vi "dataAcq_get_spectrum_trace.vi"(0 "reference":refnum<class "OSA.lvclass">, 2 "spectrum trace index":u32, 5 "error in (no error)":errorcluster, 7 "spectrum trace set name":string, 9 "parameter trace set comment":string) -> (14 "duplicate reference":refnum<class "OSA.lvclass">, 19 "error out":errorcluster)   [LabVIEW 2010, in "OSA.lvclass"]
doc: "Reads data from spectrometer and updates a spectrum trace Y array, X is either equidistant, (x min and max), or a full X-array - see traces_xValueFormat.vi. The trace data buffer is allocated by FTSLib.dll during labview driver initialisation.\n\nX: periods/cm\nY: mW absolute pwr, (pwr/resolution)"
uses:
  OSA.lvclass
  typeDef/trace_properties_string.ctl
  OSA20X_misc.lvlib
  FTSLib.dll
panel:
  in  "parameter":T1=enum."name [max 32]"
  in  "length":u32
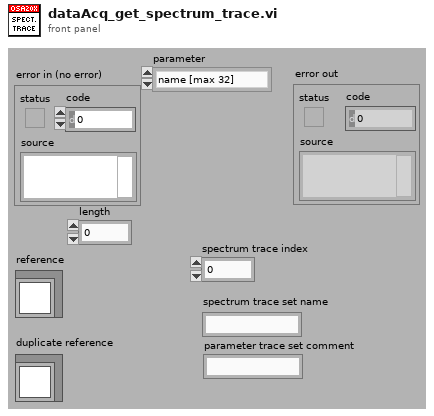
[diagram p1: front panel]
types:
  T1 = typedef "OSA.lvclass/trace_properties_string.ctl" = enum16{"interferometerSerial [max 32]", "name [max 32]", "comment [max 128]", "source [max 24]", "instr_operator [max 24]", "instr_model_str [max 24]", "all_stringParameters"}
  T2 = typedef "OSA.lvclass/ObjectAttributes.ctl" = cluster{"Stop":bool, "dataType":T3, "spectrometerIdx":u16, "buffer size interferogram":i32, "interferogram":cluster{"new":bool, "plot_x_ min":sgl, "plot_x_max":sgl, "plot_y_min":sgl, "plot_y_max":sgl, "Graph Intrfrgrm":T4, "timeStamp":u32, "signal (%)":dbl, "traces":cluster{"idx":u32, "broadBand":bool, "monoChromatic":bool, "peakToPeakSignal":dbl, "peakToPeakPos":dbl}[], "traces idx last":i32}, "spectrum":cluster{"new":bool, "plot_x_min":sgl, "plot_x_max":sgl, "plot_unit_x":T5, "plot_unit_y":T6, "plot_y_min":sgl, "plot_y_max":sgl, "Graph Spectrum":T4, "timeStamp":u32, "X_VAL_OPTIONS":enum16{"MIN_MAX", "ARRAY"}, "traces":cluster{"idx":u32}[], "traces idx last":i32}, "Thorlabs_OSA_64.lvclass:queue_action.ctlqueue ref":refnum<queue>, "action":T7, "plot zoom step":dbl, "buffer semaphore":T8, "acq stopped":bool, "dataType active":T3, "temperature (degr C)":sgl, "pressure (hPa)":sgl, "rel humidity (%)":sgl, "settings":cluster{"resolution":T9, "sensitivity":T10, "Average":bool, "average nr":u32, "apodisation":T11, "acq delay (ms)":u32, "airMesure":T12, "wmtr on":bool, "intfgrm_smooth_width":u16, "intfgrm_smooth_nrOfPasses":u16, "intfgrm_smooth":T13, "phaseCorrection":T14, "zeroFill":u8, "spectr_smooth":T13, "spectr_smooth_width":u16, "spectr_smooth_nrOfPasses":u16, "resolution (/cm)":sgl, "REF wavelength, (nm)":dbl, "gain_idx":u16, "gainAuto":bool, "gain_relative":dbl, "PD sensitivity mode":T15, "PD senseMode implemented":bool, "SensorTemperature implemented":bool, "SensorPressure implemented":bool, "SensorHumidity implemented":bool}, "peaks position":sgl[], "peaks width":sgl[], "peaks height":sgl[], "peaks max nr":u32, "peaks latest nr":i32, "peaks new":bool, "power":dbl, "power new":bool, "path":string, "wavelength (WNr)":dbl, "wavelength new":bool, "buffer size spectrum":i32, "status":string, "VI reference":refnum<vi>, "funcPointer":u64, "libraryPointer":u64, "singleAcquisition":bool, "coherenceLength (cm)":dbl, "coherenceLength new":bool, "spectrometer model":string, "spectrometer serial nr":string, "peaks thld left":sgl[], "peaks thld right":sgl[], "coherenceLength error (cm)":dbl, "ADC bits":u16, "peaks position centroid":sgl[], "peaks height centroid":sgl[], "OSA series":T16, "channel index spectrum":u16, "spectrometer rangeLow, (/cm)":dbl, "spectrometer rangeHigh, (/cm)":dbl, "channel index interferogram":u16}
  T3 = typedef "OSA.lvclass/acq_dataType.ctl" = enum16{"none", "interferogram", "spectrum"}
  T4 = typedef "OSA.lvclass/graph_intensity.ctl" = refnum<vi>
  T5 = typedef "OSA.lvclass/spectrum_x_unit.ctl" = enum16{"wavenr/cm", "THz", "eV", "nm_air", "nm_vac"}
  T6 = typedef "OSA.lvclass/y_unit.ctl" = enum16{"ADC counts", "dBm pwr absolute", "dBm pwr density", "mW pwr absolute", "mW pwr density"}
  T7 = typedef "OSA.lvclass/queue_action.ctl" = enum16{"none", "stop", "GUI_plotInterferogram", "GUI_plotSpectrum", "GUI_plotInterferogramRescale", "GUI_plotSpectrumRescale", "GUI_plotInterferogramReset", "GUI_plotSpectrumReset", "GUI_plotInterferogramAutoScaleY", "GUI_plotSpectrumAutoScaleY", "GUI_plotInterferogramZoomOut", "GUI_plotSpectrumZoomOut", "GUI_plotInterferogramPane", "GUI_plotSpectrumPane", "GUI_plotInterferogramZoomMouse", "GUI_plotSpectrumZoomMouse", "ENVIRONMENT temperature", "ENVIRONMENT pressure", "MODE_resolution set", "MODE_resolution get", "MODE_sensitivity set", "MODE_sensitivity get", "MODE_PDTemperature set", "MODE_PDTemperature get", "REBOOT/RESET firmware", "ACQASYNC_acquireSingleSpectrum", "ACQASYNC_continuous start", "ACQASYNC_continuous stop\n", "ACQASYNC_get last interferogram", "ACQASYNC_get last spectrum", "ACQASYNC_get last waveNr", "ACQOPT_interferogram smoothing set", "ACQOPT_interferogram smoothing get", "ACQOPT_spectrum smoothing set", "ACQOPT_spectrum smoothing get", "ACQOPT_apodisation type set", "ACQOPT_apodisation type get", "ACQOPT_phase correction type set", "ACQOPT_phase correction type get", "ACQOPT_acqIntervall_set", "ACQOPT_acqIntervall_get", "ACQOPT_average spectrum set", "ACQOPT_average spectrum get", "ACQOPT_rolling average set", "ACQOPT_rolling average get", "ACQOPT_zero fill factor set", "ACQOPT_zero fill factor get", "ACQOPT_cycle counting set", "ACQOPT_cycle counting get", "ACQOPT_air measure option set", "ACQOPT_air measure option get", "ACQOPT_gainLevel auto get", "ACQOPT_gainLevel auto set", "ACQOPT_gainLevel get", "ACQOPT_gainLevel set", "ACQOPT_getAll", "INSTRUMENT_PROPERTY_range_WaveNr_min", "INSTRUMENT_PROPERTY_range_WaveNr_max", "INSTRUMENT_PROPERTY_reference_wavelength_cm^-1", "INSTRUMENT_PROPERTY_samplesPerRefPeriod", "INSTRUMENT_PROPERTY_resolution_waveNrPercm", "INSTRUMENT_PROPERTY_availableGainLevels", "INSTRUMENT_PROPERTY_status", "CONVERT", "ANALYSE_POWER", "ANALYSE_PEAKS", "ANALYSE_WAVELENGTH", "ANALYSE_SPECTRUM", "ANALYSE_INTERFEROGRAM", "ANALYSE_COHERENCE_LENGTH", "MATH", "MATH_power", "MATH_peaks", "FILE", "miscellaneous"}
  T8 = typedef "Semaphore RefNum" = refnum<k1>
  T9 = typedef "OSA.lvclass/resolution.ctl" = enum16{"low", "high"}
  T10 = typedef "OSA.lvclass/sensitivityMode.ctl" = enum16{"low", "low medium", "high medium", "high"}
  T11 = typedef "OSA.lvclass/apodisation.ctl" = enum16{"NONE", "NORTON_BEER_WEAK", "NORTON_BEER_MEDIUM", "NORTON_BEER_STRONG", "TRIANGULAR", "COSINE", "HANN", "HAMMING", "BLACKMANHARRIS3", "BLACKMANHARRIS4", "GAUSSIAN"}
  T12 = typedef "OSA.lvclass/airMeasure.ctl" = enum16{"TEMPERATURE", "PRESSURE"}
  T13 = typedef "OSA.lvclass/smoothing.ctl" = enum16{"NONE", "BINOMIAL", "SAVITSKY_GOLAY", "FOURIER", "MOVING_AVERAGE", "GAUSSIAN"}
  T14 = typedef "OSA.lvclass/phaseCorrection.ctl" = enum16{"NONE", "MERTZ", "FORMAN", "MERTZ_FILE", "FORMAN_FILE", "FUTURE COMP."}
  T15 = typedef "OSA.lvclass/PDTemperatureMode.ctl" = enum16{"cool: better sensitivity/noise floor", "warm: extended wl range"}
  T16 = typedef "OSA.lvclass/OSA_series.ctl" = enum16{"OSA200", "OSA300", "UNKNOWN"}
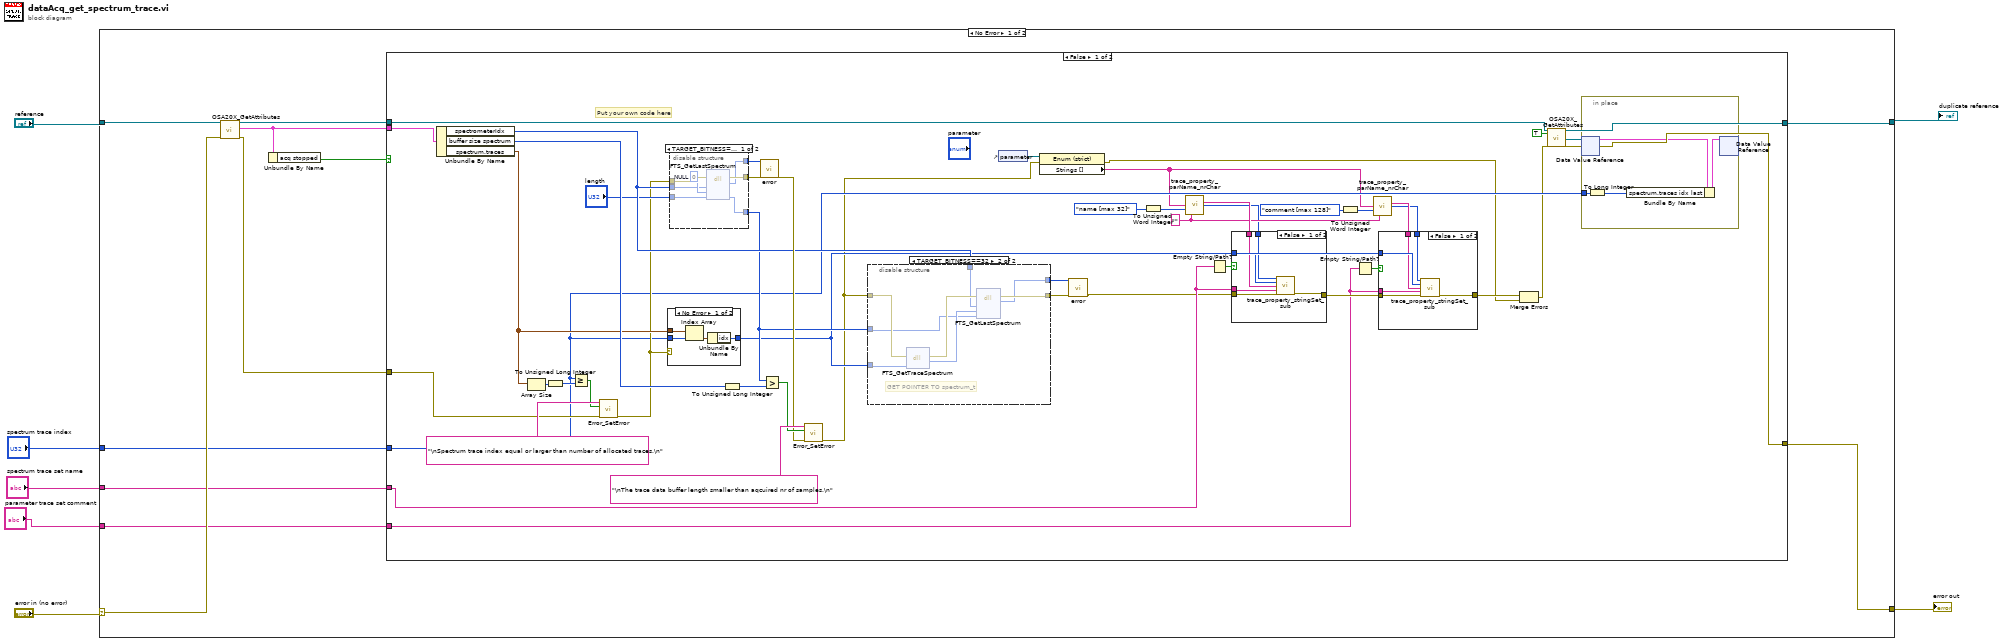
[diagram p0: block diagram]
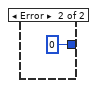
[diagram p4: hidden frame]
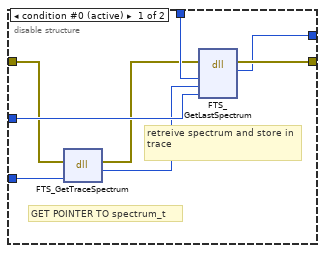
[diagram p5: hidden frame]
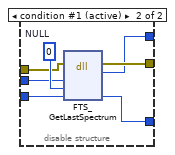
[diagram p6: hidden frame]
diagram:
  n1 = case shown="No Error" "error in (no error)" {
    selector: "error in (no error)" -> [w17 w123]
    tunnel: [w15 w123] -> w6
    tunnel: "reference" -> [w18 w122]
    tunnel: [w16 w122] -> w4
    tunnel: "spectrum trace index" -> [w12 _]
    tunnel: "spectrum trace set name" -> [w9 _]
    tunnel: "parameter trace set comment" -> [w8 _]
    frame No Error {
      n2 = call "OSA20X_GetAttributes.vi"("reference in"=w18, "error in (no error)"=w17) -> ("reference out"=w14:refnum<class "OSA.lvclass">, "Data"=w13:T2, "error out"=w11:errorcluster)  [unwired: 14 in, 1 out]
      n3 = Unbundle By Name(w13) -> ("acq stopped"=w10:bool)
      n4 = case shown="False" w10 {
        tunnel: w13 -> [w50 _]
        tunnel: w14 -> [w31 w121]
        tunnel: [w63 w121] -> w16
        tunnel: [w62 w120] -> w15
        tunnel: w11 -> [w46 w120]
        tunnel: w12 -> [w37 _]
        tunnel: w9 -> [w41 _]
        tunnel: w8 -> [w39 _]
        frame False {
          w22 = "" ("all string")
          # "Put your own code here"
          n5 = Unbundle By Name(w50) -> ("spectrometerIdx"=w55:u16, "buffer size spectrum"=w64:i32, "spectrum.traces"=w44:cluster{"idx":u32}[])
          n6 = Array Size(array=w44) -> (size(s)=w49:i32)
          n7 = To Unsigned Long Integer(number=w49) -> (unsigned 32bit integer=w48:u32)
          n8 = Greater Or Equal?(x=w37, y=w48) -> (x >= y?=w45:bool)
          n9 = call "Error_SetError.vi"("error in"=w46, "status (true)"=w45, "source(\"\")"="\nSpectrum trace index equal or larger than number of allocated traces.\n" ("source(\"\")")) -> ("error out"=w43:errorcluster)  [unwired: 4 in]
          n10 = case shown="No Error" w43 {
            tunnel: w44 -> [w84 _]
            tunnel: w37 -> [w83 _]
            tunnel: [w81 u32 0 ("idx")] -> w33
            frame No Error {
              n11 = Index Array(array=w84, index=w83) -> (element=w82:cluster{"idx":u32})
              n12 = Unbundle By Name(w82) -> ("idx"=w81:u32)
            }
            frame Error {
            }
          }
          n13 = disable-structure shown="TARGET_BITNESS==32" {
            disable-tunnel: w55 -> [w104 w113]
            disable-tunnel: [w102 w110] -> w52
            disable-tunnel: [w108 w114] -> w58
            disable-tunnel: "length" -> [w106 w112]
            disable-tunnel: [w103 w111] -> w56
            disable-tunnel: w43 -> [w107 w109]
            frame condition #0 {
              w105 = u32 0  # NULL
              n14 = dll-call lib="FTSLib.dll" fn="FTS_GetLastSpectrum"(error in=w107, "spectrIdx"=w104, "spec"=w105, "length"=w106) -> (error out=w108:errorcluster, "return type"=w103:i32, "length"=w102:u32)  [unwired: 4 in, 1 out]
            }
            frame condition #1 (active) {
              w115 = u64 0  # NULL
              n15 = dll-call lib="FTSLib.dll" fn="FTS_GetLastSpectrum"(error in=w109, "spectrIdx"=w113, "spec"=w115, "length"=w112) -> (error out=w114:errorcluster, "return type"=w111:i32, "length"=w110:u32)  [unwired: 4 in, 1 out]
            }
          }
          n16 = To Unsigned Long Integer(number=w64) -> (unsigned 32bit integer=w61:u32)
          n17 = call "error.vi"("result code"=w56, "error in (no error)"=w58) -> ("error out"=w57:errorcluster)  [unwired: 15 in, 2 out]
          n18 = Greater?(x=w52, y=w61) -> (0:w65:bool)
          n19 = call "Error_SetError.vi"("error in"=w57, "status (true)"=w65, "source(\"\")"="\nThe trace data buffer length smaller than aqcuired nr of samples.\n" ("source(\"\")")) -> ("error out"=w30:errorcluster)  [unwired: 4 in]
          n20 = disable-structure shown="TARGET_BITNESS==32" {
            disable-tunnel: w55 -> [w93 w94]
            disable-tunnel: w30 -> [w87 w98]
            disable-tunnel: [w92 w96] -> w54
            disable-tunnel: [w91 w95] -> w53
            disable-tunnel: w52 -> [w90 w97]
            disable-tunnel: w33 -> [w89 w99]
            frame condition #0 (active) {
              # "retreive spectrum and store in trace"
              # "GET POINTER TO spectrum_t"
              n21 = dll-call lib="FTSLib.dll" fn="FTS_GetTraceSpectrum"(error in=w87, "traceIdx"=w89) -> (error out=w86:errorcluster, "spectrum_t_pointer"=w88:u64)  [unwired: 3 in, 1 out]
              n22 = dll-call lib="FTSLib.dll" fn="FTS_GetLastSpectrum"(error in=w86, "spectrIdx"=w93, "spectrum_t_pointer"=w88, "length"=w90) -> (error out=w92:errorcluster, "return type"=w91:i32)  [unwired: 5 in, 1 out]
            }
            frame condition #1 {
              # "GET POINTER TO spectrum_t"
              n23 = dll-call lib="FTSLib.dll" fn="FTS_GetTraceSpectrum"(error in=w98, "traceIdx"=w99) -> (error out=w100:errorcluster, "spectrum_t_pointer"=w101:u32)  [unwired: 3 in, 1 out]
              n24 = dll-call lib="FTSLib.dll" fn="FTS_GetLastSpectrum"(error in=w100, "spectrIdx"=w94, "spectrum_t_pointer"=w101, "length"=w97) -> (error out=w96:errorcluster, "return type"=w95:i32)  [unwired: 5 in, 1 out]
            }
          }
          n25 = control-ref of="parameter"() -> (w36:refnum<vi>)
          n26 = property class="Enum (strict)"(reference=w36, error in=w30) -> (error out=w28:errorcluster, "Strings []"=w23:string[])  [unwired: 1 out]
          n27 = call "error.vi"("result code"=w53, "error in (no error)"=w54) -> ("error out"=w32:errorcluster)  [unwired: 15 in, 2 out]
          n28 = To Unsigned Word Integer(number=trace_properties_string."name [max 32]" ("parameter")) -> (unsigned 16bit integer=w26:u16)
          n29 = call "trace_property_parName_nrChar.vi"("Strings enum"=w23, "Value enum"=w26, "all string"=w22) -> ("parameter names"=w24:string[], "char nr max"=w19:i32[])  [unwired: 11 in]
          n30 = Empty String/Path?(string/path=w41) -> (empty?=w40:bool)
          n31 = case shown="False" w40 {
            tunnel: [w78 w80] -> w42
            tunnel: w32 -> [w79 w80]
            tunnel: w41 -> [w75 _]
            tunnel: w24 -> [w77 _]
            tunnel: w33 -> [w76 _]
            tunnel: w19 -> [w74 _]
            frame False {
              n32 = call "trace_property_stringSet_sub.vi"("char nr max"=w74, "trace idx global"=w76, "parameter_name"=w77, "parameter_value"=w75, "error in (no error)"=w79) -> ("error out"=w78:errorcluster)  [unwired: 10 in]
            }
            frame True {
            }
          }
          n33 = To Unsigned Word Integer(number=trace_properties_string."comment [max 128]" ("parameter")) -> (unsigned 16bit integer=w25:u16)
          n34 = Empty String/Path?(string/path=w39) -> (empty?=w38:bool)
          n35 = call "trace_property_parName_nrChar.vi"("Strings enum"=w23, "Value enum"=w25, "all string"=w22) -> ("parameter names"=w21:string[], "char nr max"=w20:i32[])  [unwired: 11 in]
          n36 = case shown="False" w38 {
            tunnel: w42 -> [w72 w73]
            tunnel: [w71 w73] -> w29
            tunnel: w39 -> [w69 _]
            tunnel: w33 -> [w70 _]
            tunnel: w21 -> [w68 _]
            tunnel: w20 -> [w67 _]
            frame False {
              n37 = call "trace_property_stringSet_sub.vi"("char nr max"=w67, "trace idx global"=w70, "parameter_name"=w68, "parameter_value"=w69, "error in (no error)"=w72) -> ("error out"=w71:errorcluster)  [unwired: 10 in]
            }
            frame True {
            }
          }
          n38 = Merge Errors(w29, w28) -> (w27:errorcluster)
          n39 = call "OSA20X_GetAttributes.vi"("reference in"=w31, "OnlyGetDvrReference(False)"=TRUE, "error in (no error)"=w27) -> ("reference out"=w63:refnum<class "OSA.lvclass">, "DataRef"=w59:refnum<data-value>, "error out"=w62:errorcluster)  [unwired: 13 in, 1 out]
          n40 = in-place {
            in-place-border: w37 -> [w118]
            n41 = in-place-dvr #1(w59) -> (w119:T2)  [unwired: 1 out]
            n42 = To Long Integer(number=w118) -> (32bit integer=w116:i32)
            n43 = Bundle By Name(cluster=w119, "spectrum.traces idx last"=w116) -> (w117:T2)
            n44 = in-place-dvr #1(w117) -> ()  [unwired: 2 out]
          }
        }
        frame True {
        }
      }
    }
    frame Error {
      # "Error"
    }
  }
  "error out" <- w6
  "duplicate reference" <- w4
